vi "SensorLoop.vi"   [LabVIEW 2017]
uses:
  <userlib>/836-Library/System/QCP_V2/QCPSupportCode/QCP_GetDbl.vi
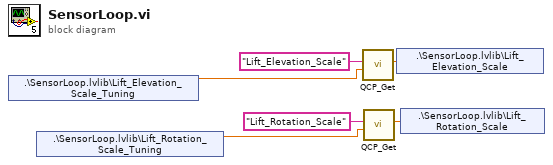
[diagram p0: block diagram]
diagram:
  n1 = shared-variable ".\\SensorLoop.lvlib\\Lift_Elevation_Scale_Tuning"() -> (w1:dbl)  [unwired: 1 in, 1 out]
  n2 = shared-variable ".\\SensorLoop.lvlib\\Lift_Rotation_Scale_Tuning"() -> (w2:dbl)  [unwired: 1 in, 1 out]
  n3 = call-poly <userlib>:"QCP_Get.vi"("Tuning Value"=w1, "Value Name"="Lift_Elevation_Scale") -> ("Value"=w5:dbl)  [unwired: 7 in, 2 out]
  n4 = call-poly <userlib>:"QCP_Get.vi"("Tuning Value"=w2, "Value Name"="Lift_Rotation_Scale") -> ("Value"=w6:dbl)  [unwired: 7 in, 2 out]
  n5 = shared-variable ".\\SensorLoop.lvlib\\Lift_Elevation_Scale"(w5) -> ()  [unwired: 1 in, 1 out]
  n6 = shared-variable ".\\SensorLoop.lvlib\\Lift_Rotation_Scale"(w6) -> ()  [unwired: 1 in, 1 out]
